vi "from_json.vi"(8 "error in":errorcluster, 11 "JSON":string) -> (0 "error out":errorcluster, 2 "User":refnum<class "User.lvclass">)   [LabVIEW 2020, in "User.lvclass"]
uses:
  User.lvclass
  User.lvclass/User.ctl
  77e552a5-7182-4905-9610-0a88d4800e8f.vi
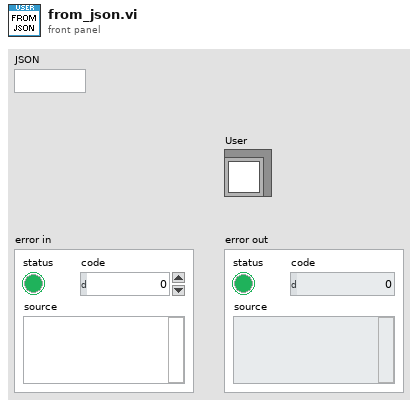
[diagram p1: front panel]
types:
  T1 = cluster{"[0]":string, "[1]":string, "[2]":string, "[3]":string, "[4]":string}
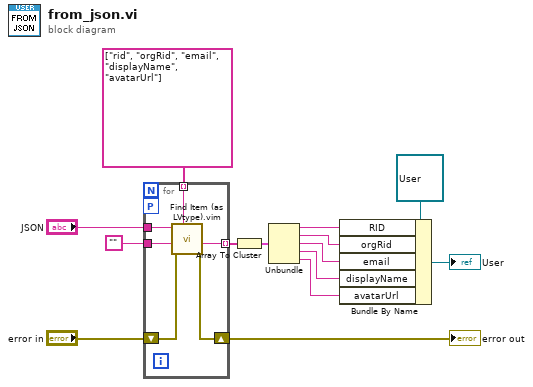
[diagram p0: block diagram]
diagram:
  n1 = for {
    tunnel: string[] ["rid", "orgRid", "email", "displayName", "avatarUrl"] -> [w20] mode=indexing
    tunnel: "JSON" -> [w19]
    tunnel: "" -> [w18]
    shift-right: [w16] -> w10
    shift-left: "error in" -> [w17]
    workers-P: _ -> [_]
    tunnel: [w15] -> w9 mode=indexing
    n2 = call "Find Item (as LVtype).vim"("$Path or Item Name"=w20, "error in (no error)"=w17, "Data Type and Default Value"=w18, "JSON"=w19) -> ("error out"=w16:errorcluster, "Data"=w15:string)  [unwired: 4 in, 2 out]
  }
  "error out" <- w10
  n3 = Array To Cluster(array=w9) -> (cluster=w8:T1)
  n4 = Unbundle(w8) -> ("[0]"=w6:string, "[1]"=w5:string, "[2]"=w3:string, "[3]"=w4:string, "[4]"=w2:string)
  n5 = Bundle By Name(cluster=refnum<class "User.lvclass"> refnum ("User"), "RID"=w6, "orgRid"=w5, "email"=w3, "displayName"=w4, "avatarUrl"=w2) -> (→"User":refnum<class "User.lvclass">)
